vi "#42_MAV_MSG_MISSION_CURRENT_DECODE.vi"(11 "mavlink_payload":u8[](array[numeric])) -> (3 "MISSION_CURRENT":T1)   [LabVIEW 2023]
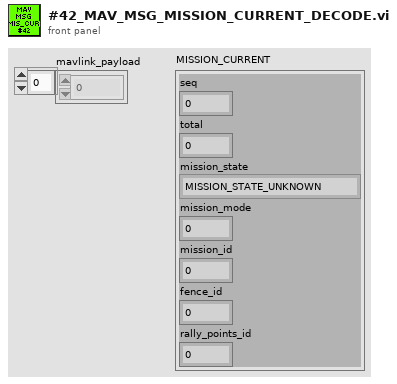
[diagram p1: front panel]
types:
  T1 = cluster{"seq":u16, "total":u16, "mission_state":enum8{"MISSION_STATE_UNKNOWN", "MISSION_STATE_NO_MISSION", "MISSION_STATE_NOT_STARTED", "MISSION_STATE_ACTIVE", "MISSION_STATE_PAUSED", "MISSION_STATE_COMPLETE"}, "mission_mode":u8, "mission_id":u32, "fence_id":u32, "rally_points_id":u32}
  T2 = enum8{"MISSION_STATE_UNKNOWN", "MISSION_STATE_NO_MISSION", "MISSION_STATE_NOT_STARTED", "MISSION_STATE_ACTIVE", "MISSION_STATE_PAUSED", "MISSION_STATE_COMPLETE"}
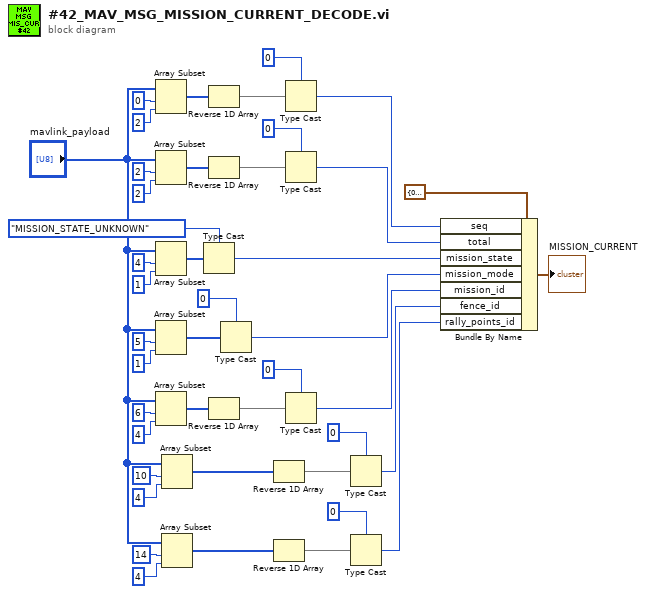
[diagram p0: block diagram]
diagram:
  n1 = Array Subset(array="mavlink_payload", index=0, length=2) -> (w43:u8[])
  n2 = Array Subset(array="mavlink_payload", index=2, length=2) -> (w35:u8[])
  n3 = Array Subset(array="mavlink_payload", index=4, length=1) -> (w27:u8[])
  n4 = Array Subset(array="mavlink_payload", index=5, length=1) -> (w21:u8[])
  n5 = Array Subset(array="mavlink_payload", index=6, length=4) -> (w19:u8[])
  n6 = Array Subset(array="mavlink_payload", index=10, length=4) -> (w13:u8[])
  n7 = Array Subset(array="mavlink_payload", index=14, length=4) -> (w7:u8[])
  n8 = Type Cast(type=T2."MISSION_STATE_UNKNOWN" ("mission_state"), x=w27) -> (*(type *) &x=w26:T2)
  n9 = Reverse 1D Array(array=w43) -> (reversed array=w42:u8[])
  n10 = Reverse 1D Array(array=w35) -> (reversed array=w34:u8[])
  n11 = Reverse 1D Array(array=w19) -> (reversed array=w18:u8[])
  n12 = Type Cast(type=u8 0 ("index"), x=w21) -> (*(type *) &x=w20:u8)
  n13 = Reverse 1D Array(array=w13) -> (reversed array=w12:u8[])
  n14 = Reverse 1D Array(array=w7) -> (reversed array=w6:u8[])
  n15 = Type Cast(type=u16 0 ("index"), x=w42) -> (*(type *) &x=w36:u16)
  n16 = Type Cast(type=u16 0 ("index"), x=w34) -> (*(type *) &x=w30:u16)
  n17 = Type Cast(type=u32 0 ("index"), x=w18) -> (*(type *) &x=w14:u32)
  n18 = Type Cast(type=u32 0 ("index"), x=w12) -> (*(type *) &x=w8:u32)
  n19 = Type Cast(type=u32 0 ("index"), x=w6) -> (*(type *) &x=w1:u32)
  n20 = Bundle By Name(cluster=T1 {"seq"=0, "total"=0, "mission_state"=enum."MISSION_STATE_UNKNOWN", "mission_mode"=0, "mission_id"=0, "fence_id"=0, "rally_points_id"=0} ("MISSION_CURRENT"), "seq"=w36, "total"=w30, "mission_state"=w26, "mission_mode"=w20, "mission_id"=w14, "fence_id"=w8, "rally_points_id"=w1) -> (→"MISSION_CURRENT":T1)
